vi "变更推送.vi"(8 "error in":errorcluster caption="错误输入（无错误）", 11 "仓库路径":path=path "E:/学习文件/Git插件/test") -> (0 "error out":errorcluster caption="错误输出", 1 "standard error":string caption="标准错误", 2 "standard output":string caption="标准输出", 3 "仓库路径":path=path "E:/学习文件/Git插件/test")   [LabVIEW 2018]
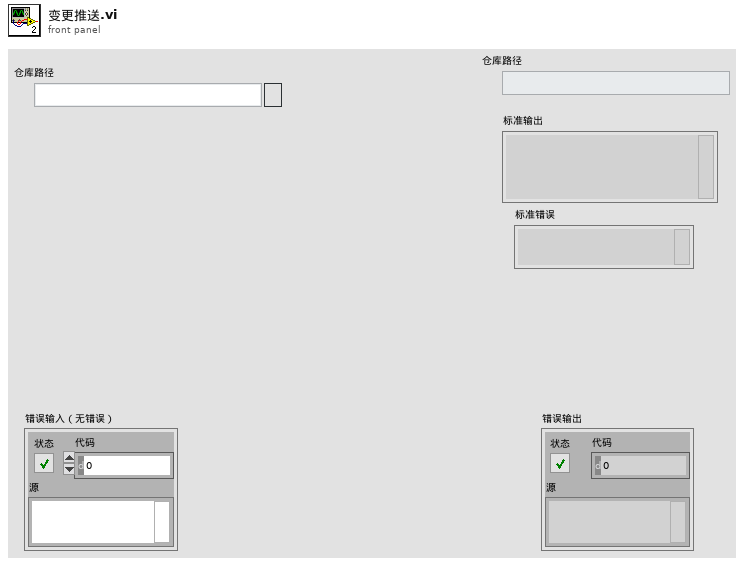
[diagram p1: front panel]
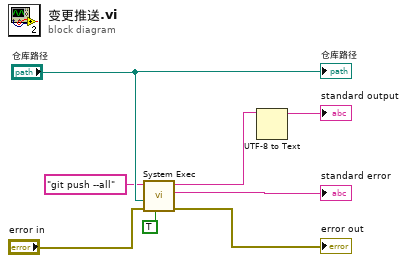
[diagram p0: block diagram]
diagram:
  n1 = call <vilib>:"System Exec.vi"("run minimized? (F)"=TRUE, "error in (no error)"="error in", "working directory"="仓库路径", "command line"="git push --all") -> ("error out"=→"error out":errorcluster, "standard error"=→"standard error":string, "standard output"=w7:string)  [unwired: 4 in, 1 out]
  n2 = UTF-8 to Text ("UTF-8至文本转换")(11:w7) -> (3:→"standard output":string)  [unwired: 2 in, 1 out]
  "仓库路径" <- "仓库路径"
